vi "test_fpga.vi"() -> ()   [LabVIEW 2013]
uses:
  <vilib>/rvi/DesktopExecutionNode/Execution/niFpgaDEN_Execute.vi
  <vilib>/rvi/DesktopExecutionNode/DesktopExecutionNode.xnode
panel:
  out "ch0 2":i16(graph)
  out "ch2 2":i16(graph)
  out "ch1 2":i16(graph)
  in  "stop":bool
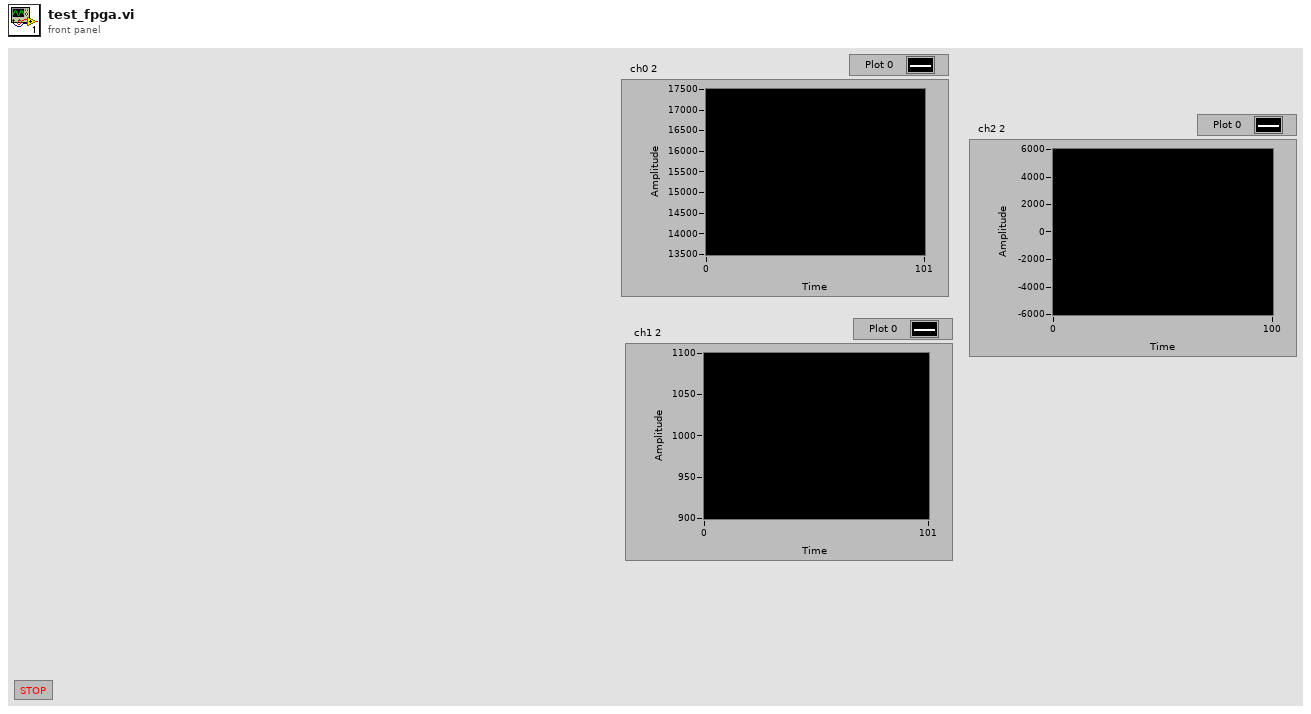
[diagram p1: front panel]
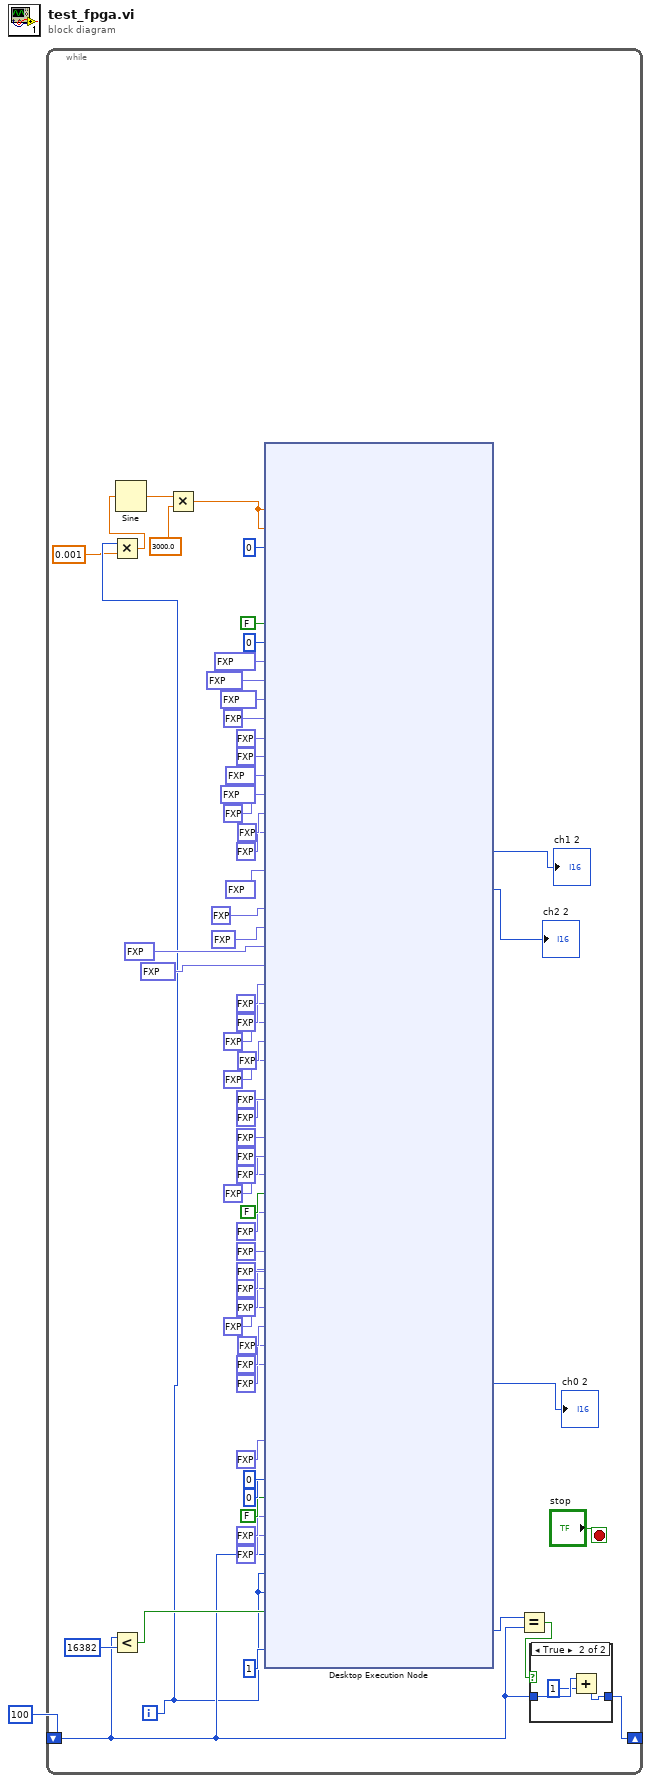
[diagram p0: block diagram]
diagram:
  n1 = while {
    shift-right: [w9] -> _
    shift-left: 100 -> [w8]
    i -> [w7]
    stop <- "stop" stop-if-true
    (unwired) fxp<+/-,16,16> 0.0 ("Setpoint 1")
    n2 = Multiply(x=w7, y=0.001) -> (x*y=w5:dbl)
    n3 = Less?(x=w8, y=16382) -> (x < y?=w13:bool)
    n4 = Sine(x=w5) -> (sin(x)=w4:dbl)
    n5 = Multiply(x=w4, y=3000.0) -> (x*y=w2:dbl)
    n6 = xnode "Desktop Execution Node"("AI0"=w2, "Connector0/AI2"=w2, "Connector0/AI1"=i16 0, "Stop"=FALSE, "Count(uSec)"=u32 0, "Lower lim 0"=fxp<+/-,32,16> -10000.0, "Upper lim 0"=fxp<+/-,32,16> 10000.0, "Dc offset 0"=fxp<+/-,32,16> 15500.0, "pg 0"=fxp<+/-,32,16> 0.0, "dg 0"=fxp<+/-,32,16> 0.0, "Lower lim 1"=fxp<+/-,32,16> 1000.0, "Upper lim 1"=fxp<+/-,32,16> -1000.0, "Dc offset 1"=fxp<+/-,32,16> 0.0, "pg 1"=fxp<+/-,32,16> 0.0, "dg 1"=fxp<+/-,32,16> 0.0, "Dc Pos 2"=fxp<+/-,32,16> 1000.0, "pg 2"=fxp<+/-,32,16> 0.0, "dg 2"=fxp<+/-,32,16> 100.0, "Upper lim 2"=fxp<+/-,32,16> 5000.0, "Lower lim 2"=fxp<+/-,32,16> -5000.0, "Dc offset 2"=fxp<+/-,32,16> 0.0, "1,1"=fxp<+/-,32,16> 1.0, "1, 2"=fxp<+/-,32,16> 0.0, "1, 3"=fxp<+/-,32,16> 0.0, "2, 1"=fxp<+/-,32,16> 0.0, "2, 2"=fxp<+/-,32,16> 1.0, "2, 3"=fxp<+/-,32,16> 0.0, "3, 3"=fxp<+/-,32,16> 1.0, "3, 2"=fxp<+/-,32,16> 0.0, "3, 1"=fxp<+/-,32,16> 0.0, "frequency (periods/tick)"=fxp<+,32,0> 0.0, "reset freq"=FALSE, "Drive_gain 0"=fxp<+/-,32,16> 0.0, "Zfb norm const 0"=fxp<+/-,32,16> 1.0, "Z offset 0"=fxp<+/-,32,16> 1.0, "Dc Pos 0"=fxp<+/-,32,16> 0.0, "meters per bit beam displacement 0"=fxp<+/-,32,16> 1.0, "Dc Pos 1"=fxp<+/-,32,16> 1.0, "Drive_gain 1"=fxp<+/-,32,16> 0.0, "Z offset 1"=fxp<+/-,32,16> 1.0, "meters per bit beam displacement 1"=fxp<+/-,32,16> 1.0, "Zfb norm const"=fxp<+/-,32,16> 0.0, "Arb gain (ch2)"=u16 0 ("RMS 1 (bits)"), "Arb gain (ch1)"=u16 0 ("RMS 0 (bits)"), "apply corrections"=FALSE, "meters per measured bit 1"=fxp<+/-,32,16> 1.0, "meters per measured bit 0"=fxp<+/-,32,16> 1.0, "write_address"=w8, "data_buffer_1"=w7, "data_buffer2"=w7, "ready_to_write"=w13, "Arb steps per cycle"=u16 1) -> ("fb+dc+drive_1"=→"ch1 2":i16, "fb +dc_2"=→"ch2 2":i16, "fb+dc+drive_0"=→"ch0 2":i16, "written_address"=w11:u32)  [unwired: 1 in, 6 out]
    n7 = Equal?(x=w11, y=w8) -> (x = y?=w10:bool)
    n8 = case shown="True" w10 {
      tunnel: [w64 w65] -> w9
      tunnel: w8 -> [w64 w67]
      frame False {
      }
      frame True {
        n9 = Add(x=w67, y=1) -> (x+y=w65:i32)
      }
    }
  }
